vi "setPath.vi"(8 "error in (no error)":errorcluster, 10 "Path":path=path "C:/Users/Administrator/Desktop/Crete/Data/2014/1411/141126/Scripts/Instrument Scripts/Dio64.csv", 11 "FileReader in":refnum<class "FileReader.lvclass">) -> (0 "error out":errorcluster, 3 "FileReader out":refnum<class "FileReader.lvclass">)   [LabVIEW 2011, in "Tools.lvlib" / "Filing.lvlib" / "FileReader.lvclass"]
uses:
  FileReader.lvclass
  FileReader.lvclass/FileReader.ctl
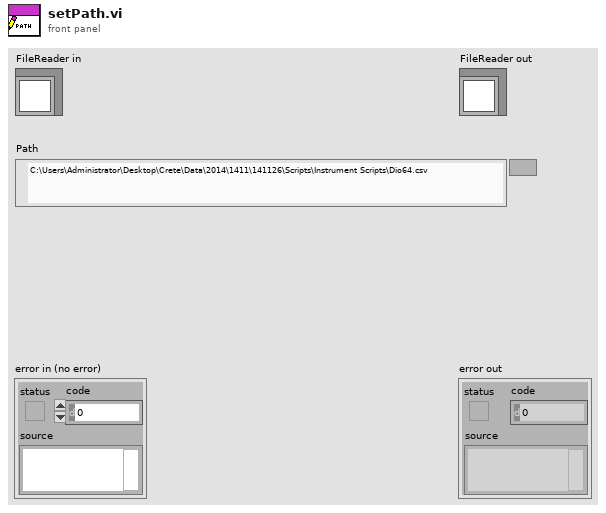
[diagram p1: front panel]
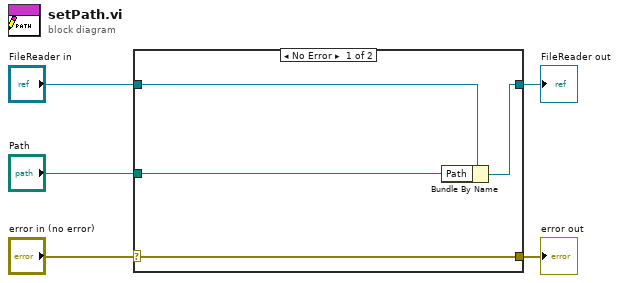
[diagram p0: block diagram]
diagram:
  n1 = case shown="No Error" "error in (no error)" {
    selector: "error in (no error)" -> [w9 w10]
    tunnel: [w9 w10] -> w4
    tunnel: [w7 w11] -> w2
    tunnel: "FileReader in" -> [w8 w11]
    tunnel: "Path" -> [w6 _]
    frame No Error {
      n2 = Bundle By Name(cluster=w8, "Path"=w6) -> (w7:refnum<class "FileReader.lvclass">)
    }
    frame Error {
    }
  }
  "error out" <- w4
  "FileReader out" <- w2
